vi "Print XML Recursive Priv.vi"(0 "Tree Dictionary In":variant, 2 "Data Types Dict":variant, 5 "DOM Doc In":refnum<k20>, 7 "Child IDs":string[](array[string]), 9 "Parent Node In":refnum<k20>, 11 "error in":errorcluster) -> (4 "Tree Dictionary Out":variant, 6 "DOM Doc Out":refnum<k20>, 10 "Parent Node Out":refnum<k20>, 15 "error out":errorcluster)   [LabVIEW 2016, in "Tree Manager.lvclass"]
uses:
  Tree Manager.lvclass
  <vilib>/xml/Close Reference(Node).vi
  <vilib>/xml/NI_XML.lvlib
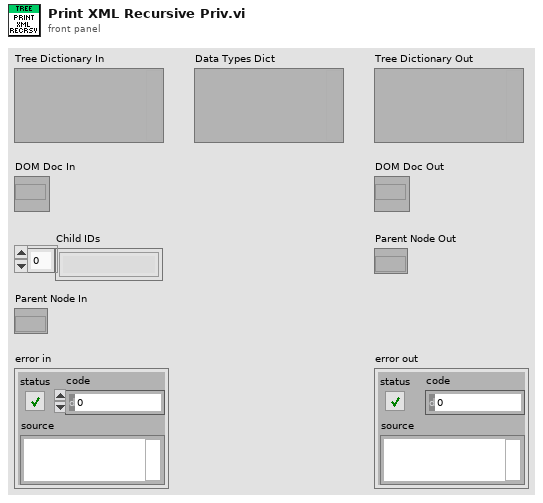
[diagram p1: front panel]
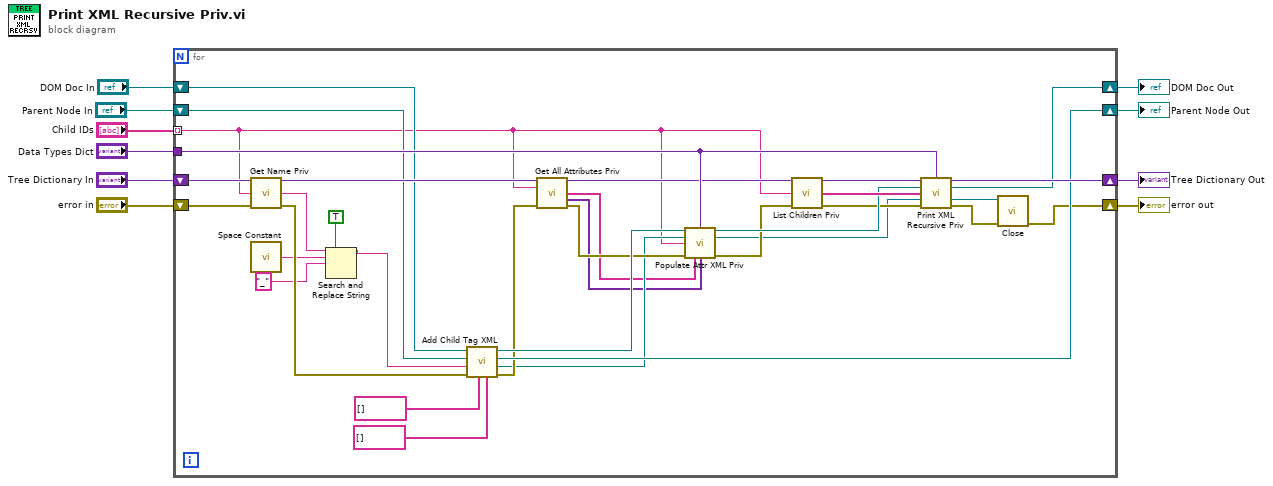
[diagram p0: block diagram]
diagram:
  n1 = for {
    tunnel: "Child IDs" -> [w18] mode=indexing
    shift-right: [w40] -> w7
    shift-left: "Tree Dictionary In" -> [w43]
    shift-right: [w29] -> w10
    shift-left: "error in" -> [w42]
    tunnel: "Data Types Dict" -> [w38]
    shift-right: [w37] -> w3
    shift-left: "DOM Doc In" -> [w35]
    shift-right: [w33] -> w1
    shift-left: "Parent Node In" -> [w32]
    n2 = call "Get Name Priv.vi"("Tree Dictionary"=w43, "Unique ID"=w18, "error in"=w42) -> ("Tree Dictionary Out"=w44:variant, "Name"=w17:string, "error out"=w28:errorcluster)  [unwired: 10 in]
    n3 = call <vilib>:"Space Constant.vi"() -> ("String"=w16:string)
    n4 = Search and Replace String(replace all?=TRUE ("replace all? (F)"), input string=w17, search string=w16, replace string="_") -> (result string=w13:string)  [unwired: 4 in, 3 out]
    n5 = call "Add Child Tag XML.vi"("Values"=string[] [], "Names"=string[] [], "Error In"=w28, "Tag Name"=w13, "Parent Node"=w32, "DOM In"=w35) -> ("Error Out"=w27:errorcluster, "Child Node"=w22:refnum<k20>, "Parent Node"=w33:refnum<k20>, "DOM Out"=w34:refnum<k20>)  [unwired: 2 in]
    n6 = call "Get All Attributes Priv.vi"("Tree Dictionary In"=w44, "Unique ID"=w18, "error in"=w27) -> ("Tree Dictionary Out"=w25:variant, "Attribute Names"=w20:string[], "Attribute Values"=w19:variant[], "error out"=w24:errorcluster)  [unwired: 9 in]
    n7 = call "Populate Attr XML Priv.vi"("DOM Doc In"=w34, "Data Types Dict"=w38, "Parent Node In"=w22, "Unique ID"=w18, "error in"=w24, "Attribute Names"=w20, "Attribute Values"=w19) -> ("DOM Doc Out"=w36:refnum<k20>, "Parent Node Out"=w21:refnum<k20>, "error out"=w23:errorcluster)  [unwired: 6 in]
    n8 = call "List Children Priv.vi"("Tree Dictionary"=w25, "Parent ID"=w18, "Error In"=w23) -> ("Tree Dictionary Out"=w41:variant, "Child IDs"=w39:string[], "Error Out"=w26:errorcluster)  [unwired: 10 in]
    n9 = call "Print XML Recursive Priv.vi"("Tree Dictionary In"=w41, "Data Types Dict"=w38, "DOM Doc In"=w36, "Child IDs"=w39, "Parent Node In"=w21, "error in"=w26) -> ("Tree Dictionary Out"=w40:variant, "DOM Doc Out"=w37:refnum<k20>, "Parent Node Out"=w31:refnum<k20>, "error out"=w30:errorcluster)  [unwired: 6 in]
    n10 = call-poly <vilib>:"Close.vi"("error in (no error)"=w30, "node"=w31) -> ("error out"=w29:errorcluster)  [unwired: 7 in]
  }
  "error out" <- w10
  "Tree Dictionary Out" <- w7
  "DOM Doc Out" <- w3
  "Parent Node Out" <- w1
